vi "Duplicate Test Executive.vi"(8 "error in (no error)":errorcluster, 11 "Test Executive in":refnum<class "Test Executive.lvclass">) -> (0 "error out":errorcluster, 3 "Test Executive out":refnum<class "Test Executive.lvclass">, 5 "Test ID out":string)   [LabVIEW 2020, in "Test Executive.lvlib" / "Test Executive.lvclass"]
uses:
  <vilib>/gpm_packages/@cs/test-executive/Source/Test Executive/TestExecutive/Test Executive.lvclass
  <vilib>/gpm_packages/@cs/test-executive/Source/Test Executive/TestExecutive/Test Executive.lvclass/Test Executive.ctl
  <vilib>/gpm_packages/@cs/test-executive/Source/Test Executive/Executioner/Executioner.lvclass
  <vilib>/gpm_packages/@cs/linked-list/Source/Linked List/Linked List Ref/Linked List Ref.lvclass
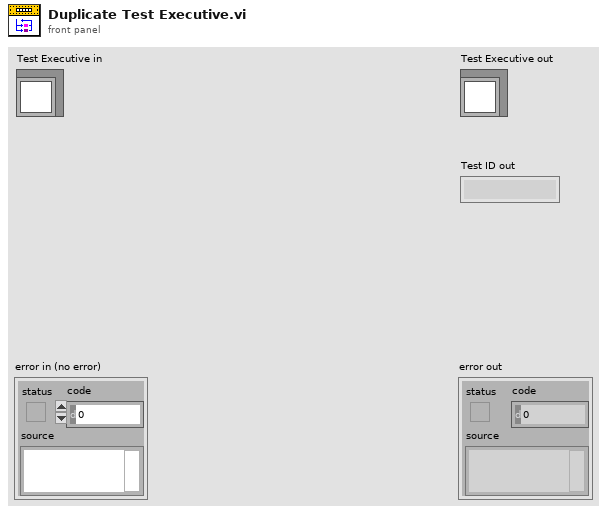
[diagram p1: front panel]
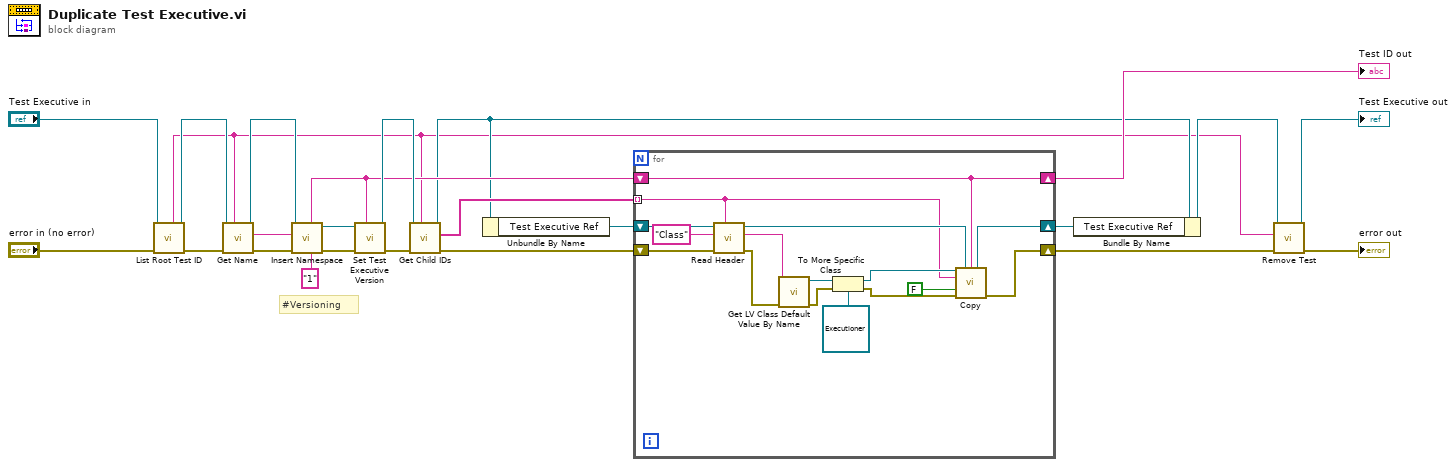
[diagram p0: block diagram]
diagram:
  # "#Versioning"
  n1 = call-dynamic "List Root Test ID.vi"("error in (no error)"="error in (no error)", "Test Executive in"="Test Executive in") -> ("error out"=w19:errorcluster, "Test Executive out"=w20:refnum<class "Test Executive.lvclass">, "Root ID"=w1:string)  [unwired: 5 in, 2 out]
  n2 = call-dynamic "Get Name.vi"("Unique ID"=w1, "error in (no error)"=w19, "Test Executive in"=w20) -> ("error out"=w14:errorcluster, "Name"=w13:string, "Test Executive out"=w16:refnum<class "Test Executive.lvclass">)  [unwired: 4 in, 2 out]
  n3 = call-dynamic "Insert Namespace.vi"("Test File Version Number"="1" ("File Version Number"), "error in (no error)"=w14, "Name"=w13, "Test Executive in"=w16) -> ("error out"=w17:errorcluster, "Test Executive out"=w15:refnum<class "Test Executive.lvclass">, "Unique ID out"=w10:string)  [unwired: 4 in, 1 out]
  n4 = call-dynamic "Set Test Executive Version.vi"("Unique ID"=w10, "error in (no error)"=w17, "Test Executive in"=w15) -> ("error out"=w12:errorcluster, "Test Executive out"=w11:refnum<class "Test Executive.lvclass">)  [unwired: 7 in]
  n5 = call-dynamic "Get Child IDs.vi"("Unique ID"=w1, "error in (no error)"=w12, "Test Executive in"=w11) -> ("error out"=w6:errorcluster, "Child IDs"=w9:string[], "Test Executive out"=w7:refnum<class "Test Executive.lvclass">)  [unwired: 6 in]
  n6 = Unbundle By Name(w7) -> ("Test Executive Ref"=w24:refnum<data-value>)
  n7 = for {
    shift-right: [w38] -> w23
    shift-left: w24 -> [w40]
    shift-right: [w39] -> w5
    shift-left: w6 -> [w28]
    tunnel: w9 -> [w26] mode=indexing
    shift-right: [w27] -> w8
    shift-left: w10 -> [w27]
    n8 = call <vilib>:"Read Header.vi"("Linked List ID"=w26, "error in (no error)"=w28, "Header Name"="Class", "Linked List Ref"=w40) -> ("error out"=w31:errorcluster, "Header Value"=w36:string, "Linked List Ref out"=w32:refnum<data-value>)  [unwired: 4 in, 1 out]
    n9 = call <vilib>:"Get LV Class Default Value By Name.vi"("error in (no error)"=w31, "class name"=w36) -> ("error out"=w30:errorcluster, "object"=w35:refnum<class>)  [unwired: 8 in]
    n10 = To More Specific Class(target class=refnum<class "Executioner.lvclass"> refnum ("Test Executive.lvlib:Executioner.lvclass"), reference=w35, error in=w30) -> (specific class reference=w33:refnum<class "Executioner.lvclass">, error out=w29:errorcluster)
    n11 = call-dynamic "Copy.vi"("Executioner in"=w33, "Linked List Ref"=w32, "New Parent ID"=w27, "Test ID"=w26, "Move?"=FALSE, "error in (no error)"=w29) -> ("Linked List Ref out"=w38:refnum<data-value>, "error out"=w39:errorcluster)  [unwired: 6 in, 2 out]
  }
  "Test ID out" <- w8
  n12 = Bundle By Name(cluster=w7, "Test Executive Ref"=w23) -> (w3:refnum<class "Test Executive.lvclass">)
  n13 = call-dynamic "Remove Test.vi"("error in (no error)"=w5, "Unique ID"=w1, "Test Executive in"=w3) -> ("error out"=→"error out":errorcluster, "Test Executive out"=→"Test Executive out":refnum<class "Test Executive.lvclass">)  [unwired: 6 in, 1 out]
